vi "Write SystemLink STR Tags.vi"(7 "Force Initialize?":bool, 8 "error in (no error)":errorcluster, 9 "timestamp":timestamp, 10 "Values":string[](array[string]), 11 "SkyLine.Refs":refnum<class "NI Skyline Tag.lvclass">[](array[class])) -> (0 "error out":errorcluster)   [LabVIEW 2019, in "Data Publishing Service.lvlib"]
uses:
  Data Publishing Service.lvlib
  <vilib>/Skyline/Tag/Wrapper/Wrapper_class/NI Skyline Tag.lvclass
  <vilib>/Skyline/Tag/Shared/typedefs/DataType.ctl
  <vilib>/Skyline/Tag/Shared/NI Skyline Tag.lvlib
  <vilib>/Skyline/Tag/Shared/typedefs/Tag Value Cluster.ctl
  <vilib>/Skyline/Configuration/Configuration_class/NI Skyline Configuration.lvclass
  <vilib>/Skyline/Tag/Wrapper/Wrapper_class/Tag Value Cluster Wrapper.ctl
  <vilib>/Skyline/Tag/Wrapper/Wrapper_class/Generate Tag Cluster (String) 2.vi
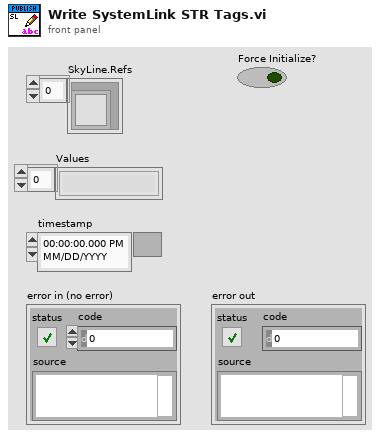
[diagram p1: front panel]
types:
  T1 = typedef "NI Skyline Tag.lvclass/Tag Value Cluster Wrapper.ctl" = cluster{"Configuration":refnum<class "NI Skyline Configuration.lvclass">, "Tag Cluster":T2}
  T2 = typedef "NI Skyline Tag.lvlib/Tag Value Cluster.ctl" = cluster{"Path":string, "Data Type":T3, "Value":string, "Time Stamp":timestamp}
  T3 = typedef "NI Skyline Tag.lvlib/DataType.ctl" = enum32{"Double", "I32", "String", "Boolean", "U64", "Timestamp"}
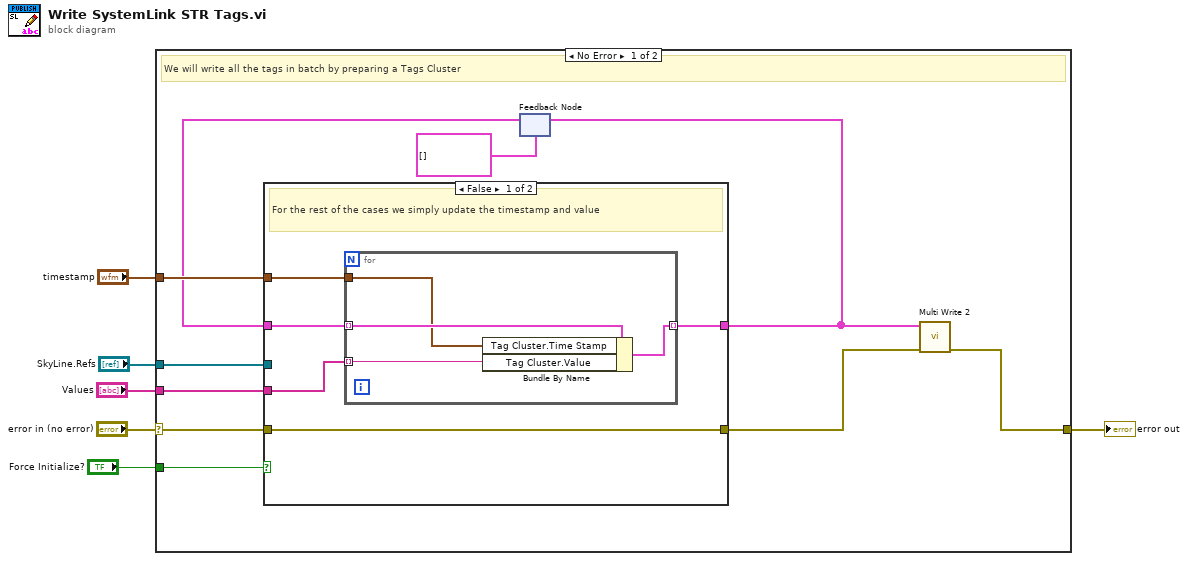
[diagram p0: block diagram]
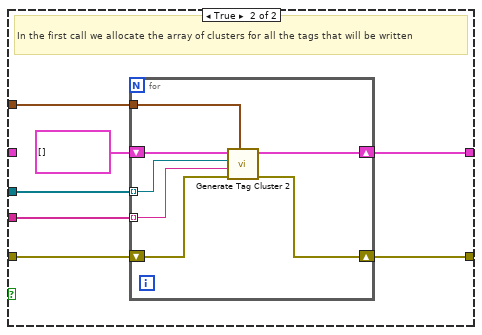
[diagram p2: hidden frame]
diagram:
  n1 = case shown="No Error" "error in (no error)" {
    selector: "error in (no error)" -> [w9 w40]
    tunnel: "SkyLine.Refs" -> [w16 _]
    tunnel: "Values" -> [w15 _]
    tunnel: "timestamp" -> [w14 _]
    tunnel: [w8 w40] -> w2
    tunnel: "Force Initialize?" -> [w7 _]
    frame No Error {
      # "We will write all the tags in batch by preparing a Tags Cluster"
      n2 = feedback #1(T1[] [] ("tag clusters in")) -> (w12:T1[])
      n3 = case shown="False" w7 {
        tunnel: w16 -> [_ w32]
        tunnel: w15 -> [w17 w31]
        tunnel: w9 -> [w21 w30]
        tunnel: w14 -> [w18 w29]
        tunnel: [w21 w28] -> w10
        tunnel: [w19 w27] -> w11
        tunnel: w12 -> [w20 _]
        frame False {
          # "For the rest of the cases we simply update the timestamp and value"
          n4 = for {
            tunnel: w20 -> [w25] mode=indexing
            tunnel: [w24] -> w19 mode=indexing
            tunnel: w18 -> [w23]
            tunnel: w17 -> [w22] mode=indexing
            n5 = Bundle By Name(cluster=w25, "Tag Cluster.Time Stamp"=w23, "Tag Cluster.Value"=w22) -> (w24:T1)
          }
        }
        frame True {
          # "In the first call we allocate the array of clusters for all the tags that will be written"
          n6 = for {
            shift-right: [w35] -> w27
            shift-left: T1[] [] ("tag clusters in") -> [w39]
            tunnel: w32 -> [w38] mode=indexing
            tunnel: w31 -> [w37] mode=indexing
            shift-right: [w33] -> w28
            shift-left: w30 -> [w36]
            tunnel: w29 -> [w34]
            n7 = call-poly <vilib>:"Generate Tag Cluster 2.vi"("time stamp"=w34, "error in (no error)"=w36, "value"=w37, "tag in"=w38, "tag clusters in"=w39) -> ("error out"=w33:errorcluster, "tag clusters out"=w35:T1[])  [unwired: 4 in, 1 out]
          }
        }
      }
      n8 = feedback-in #1(w11) -> ()
      n9 = call <vilib>:"Multi Write 2.vi"("error in (no error)"=w10, "tag clusters"=w11) -> ("error out"=w8:errorcluster)  [unwired: 9 in]
    }
    frame Error {
    }
  }
  "error out" <- w2
